vi "MC.TestLauncher.vi"() -> ()   [LabVIEW 2017, in "MC.lvclass"]
doc: "JKI State Machine Objects (SMO) 1.0.0.5\nJKI - JKI\nCopyright (c) 2016, JKI"
uses:
  MC.lvclass
  <vilib>/JKI/JKI SMO/SMO/Typedefs/SMOState --Enum.ctl
  Typedefs/Configuration--Cluster.ctl
  MC.DangwooOptron/MC.DangwooOptron.lvclass
  D:/Program Files (x86)/National Instruments/LabVIEW 2017/vi.lib/JKI/JKI SMO/SMO/SMO.lvclass
  D:/upwork/Laser Measurement Tool/Laser/project/Subsystems/MC/MC.lvclass
  D:/upwork/Laser Measurement Tool/Laser/project/Subsystems/Device/Device.lvclass
  <vilib>/JKI/JKI SMO/SMO/SMO.lvclass
  Device/Device.lvclass
panel:
  in  "Configuration":T1={"VISA Resource"="COM3"}
  out "Initialize\nResult":bool
  in  "Set Wavelength":bool
  in  "Wavelength, nm":dbl=1000.0
  out "State":T2
  out "error out":errorcluster
  in  "Stop":bool
  # "Basic SMO byRef Test Launcher"
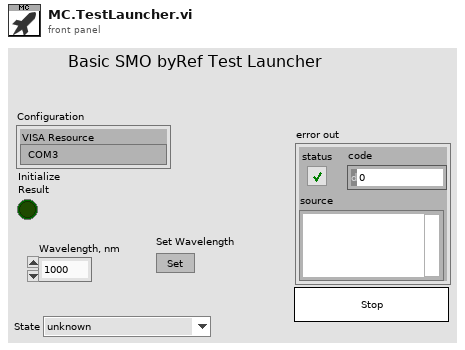
[diagram p1: front panel]
types:
  T1 = typedef "MC.lvclass/Configuration--Cluster.ctl" = cluster{"VISA Resource":string}
  T2 = typedef "SMO.lvclass/SMOState --Enum.ctl" = enum16{"unknown", "Created", "Started", "Stopped"}
  T3 = typedef "SMO.lvclass/Public Events.ctl" = cluster{"Error":refnum<user-event>, "State":refnum<user-event>, "Reserve State":refnum<user-event>}
  T4 = cluster{"Event Registration Refnum":refnum<event-registration>}
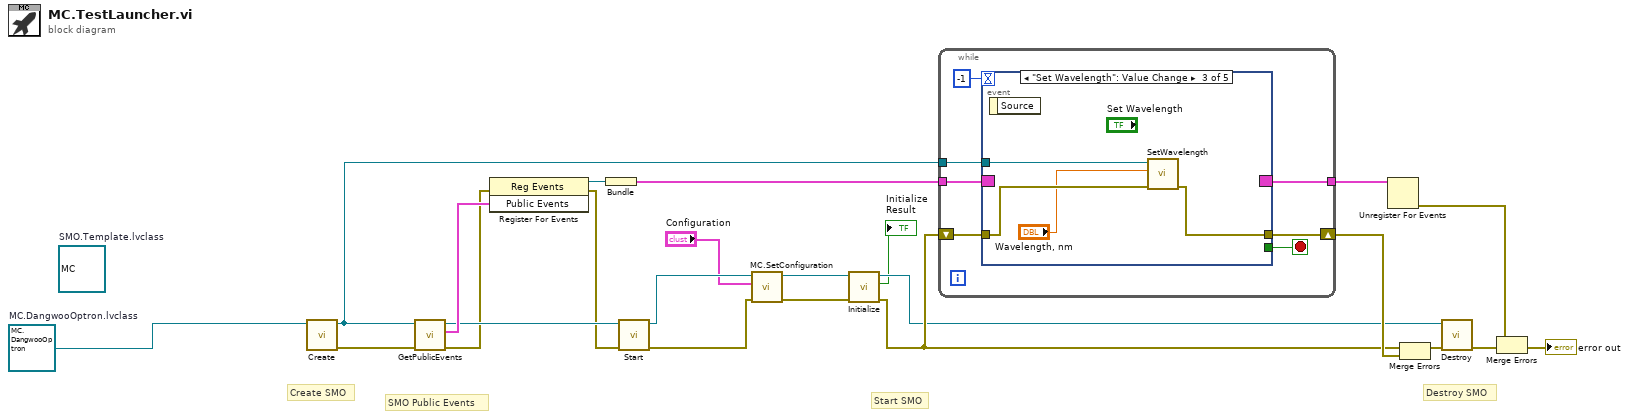
[diagram p0: block diagram]
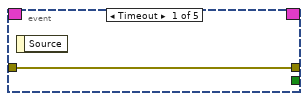
[diagram p2: hidden frame]
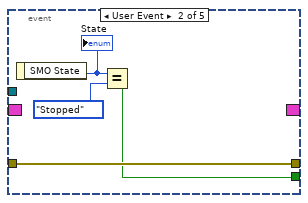
[diagram p3: hidden frame]
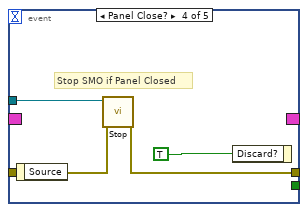
[diagram p4: hidden frame]
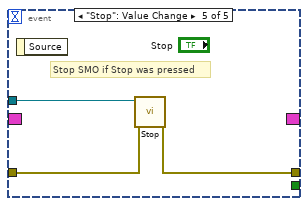
[diagram p5: hidden frame]
diagram:
  w9 = refnum<class "MC.DangwooOptron.lvclass"> refnum  # MC.DangwooOptron.lvclass
  (unwired) refnum<class "MC.lvclass"> refnum  # SMO.Template.lvclass
  # "SMO Public Events"
  # "Start SMO"
  # "Destroy SMO"
  # "Create SMO"
  n1 = call <vilib>:"Create.vi"("SMO"=w9) -> ("error out"=w10:errorcluster, "SMO out"=w16:refnum<class "MC.DangwooOptron.lvclass">)  [unwired: 8 in, 1 out]
  n2 = call <vilib>:"GetPublicEvents.vi"("error in (no error)"=w10, "SMO"=w16) -> ("error out"=w13:errorcluster, "Public Events"=w15:T3, "SMO out"=w14:refnum<class "MC.DangwooOptron.lvclass">)  [unwired: 7 in]
  n3 = register-events(error in=w13, w15) -> (reference out=w17:refnum<event-registration>, error out=w12:errorcluster)  [unwired: 1 in]
  n4 = Bundle("Event Registration Refnum"=w17) -> (w22:T4)  [unwired: 1 in]
  n5 = call <vilib>:"Start.vi"("error in (no error)"=w12, "SMO"=w14) -> ("error out"=w2:errorcluster, "SMO out"=w3:refnum<class "MC.DangwooOptron.lvclass">)  [unwired: 8 in]
  n6 = call "MC.SetConfiguration.vi"("error in (no error)"=w2, "Configuration"="Configuration", "MC"=w3) -> ("error out"=w4:errorcluster, "MC out"=w5:refnum<class "MC.DangwooOptron.lvclass">)  [unwired: 7 in]
  n7 = call "Initialize.vi"("error in (no error)"=w4, "Device in"=w5) -> ("error out"=w8:errorcluster, "Result"=→"Initialize\nResult":bool, "Device out"=w7:refnum<class "MC.DangwooOptron.lvclass">)  [unwired: 7 in]
  n8 = while {
    shift-right: [w29] -> w21
    shift-left: w8 -> [w28]
    tunnel: w22 -> [w27]
    tunnel: [w26] -> w23
    tunnel: w16 -> [w25]
    stop <- w30 stop-if-true
    n9 = event shown="[2] \"Set Wavelength\": Value Change" {
      selector: w27 -> [_ _ _ _ _]
      dyn-events: [_ _ _ _ _] -> w26
      timeout: -1 -> [_ _ _ _ _]
      tunnel: [_ w32 _ _ _] -> w30
      tunnel: w25 -> [_ _ w39 w43 w46]
      tunnel: [w31 w35 w37 w42 w45] -> w29
      tunnel: w28 -> [w31 w35 w38 w41 w44]
      event Timeout {
        n10 = event-data() -> ()  [unwired: 1 in, 1 out]
      }
      event User Event {
        n11 = event-data() -> ("SMO State"=w34:T2)  [unwired: 1 in]
        "State" <- w34
        n12 = Equal?(x=w34, y=SMOState_--Enum."Stopped") -> (x = y?=w32:bool)
      }
      event "Set Wavelength": Value Change {
        n13 = event-data() -> ()  [unwired: 1 in, 1 out]
        n14 = call "SetWavelength.vi"("error in (no error)"=w38, "Wavelength, nm"="Wavelength, nm", "MC"=w39) -> ("error out"=w37:errorcluster)  [unwired: 7 in, 1 out]
      }
      event Panel Close? {
        # "Stop SMO if Panel Closed"
        n15 = event-data() -> ()  [unwired: 1 in, 1 out]
        n16 = call <vilib>:"Stop.vi"("error in (no error)"=w41, "SMO"=w43) -> ("error out"=w42:errorcluster)  [unwired: 8 in, 1 out]
        n17 = event-data("Discard?"=TRUE ("OK")) -> ()  [unwired: 1 in, 1 out]
      }
      event "Stop": Value Change {
        # "Stop SMO if Stop was pressed"
        n18 = event-data() -> ()  [unwired: 1 in, 1 out]
        n19 = call <vilib>:"Stop.vi"("error in (no error)"=w44, "SMO"=w46) -> ("error out"=w45:errorcluster)  [unwired: 8 in, 1 out]
      }
    }
  }
  n20 = Unregister For Events(event registration refnum=w23) -> (error out=w20:errorcluster)  [unwired: 1 in]
  n21 = Merge Errors(w8, w21) -> (w11:errorcluster)
  n22 = call <vilib>:"Destroy.vi"("error in (no error)"=w11, "SMO"=w7) -> ("error out"=w18:errorcluster)  [unwired: 9 in]
  n23 = Merge Errors(w20, w18) -> (→"error out":errorcluster)
